vi "(notgoingtouse)ITXFolderToTDMS.vi"() -> ()   [LabVIEW 2016]
uses:
  <userlib>/LevyLab/LV to ITX/LVtoITX.lvclass
panel:
  in  "Add Values that were forgotten":T1(array[cluster])
  in  "Comment Values to say were extracted":string[](array[string])
  in  "Comment Values to extract":string[](array[string])
  in  "wave names to store (could wire to ITX->LV)":string[](array[string])
  out "Currrent ITX file":path
  in  "Ouput TDMS":path
  in  "Input ITX Folder":path=path "B:/SketchSET/SA03008H.20180718/21-BG+SG_Sweep+OVERNIGHT"
  # "Manually add values that were not recorded but are known"
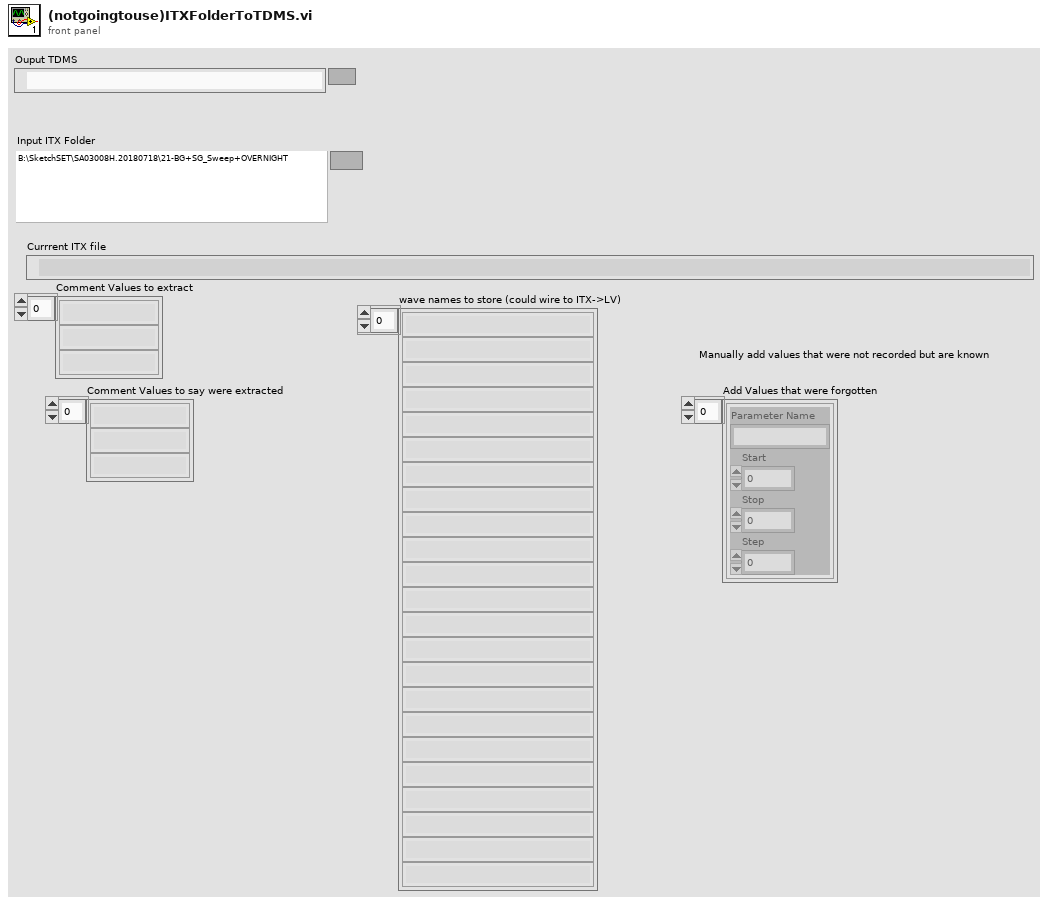
[diagram p1: front panel]
types:
  T1 = cluster{"Parameter Name":string, "Start":dbl, "Stop":dbl, "Step":dbl}[]
  T2 = enum16{"open", "open or create", "create or replace", "create", "open (read-only)"}
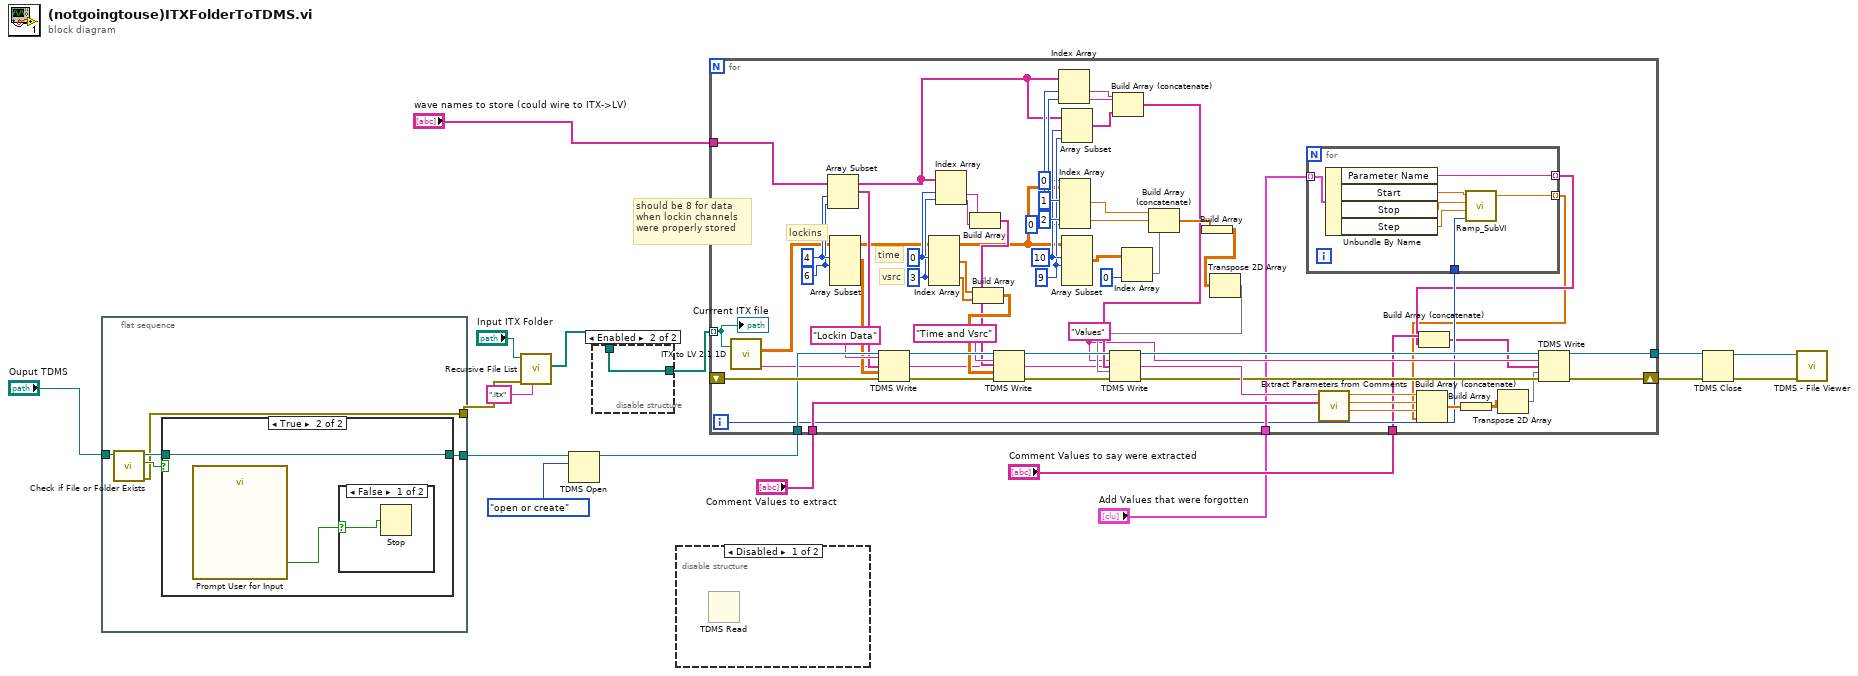
[diagram p0: block diagram]
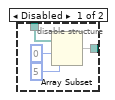
[diagram p2: hidden frame]
diagram:
  # "should be 8 for data\nwhen lockin channels\nwere properly stored"
  n1 = flat-sequence {
    tunnel: "Ouput TDMS" -> [w22]
    tunnel: [w19] -> w15
    tunnel: [w18] -> w13
    frame #0 {
      n2 = call <vilib>:"Check if File or Folder Exists.vi"("path"=w22) -> ("error out"=w18:errorcluster, "file or folder exists?"=w21:bool, "dup path"=w20:path)  [unwired: 8 in]
      n3 = case shown="True" w21 {
        tunnel: [w23 w24] -> w19
        tunnel: w20 -> [w23 w24]
        frame False {
        }
        frame True {
          n4 = call "Prompt User for Input"() -> ("Overwrite?"=w25:bool)  [unwired: 17 in, 2 out]
          n5 = case shown="False" w25 {
            selector: w25 -> [w26 _]
            frame False {
              n6 = Stop(stop? (T)=w26) -> ()
            }
            frame True {
            }
          }
        }
      }
    }
  }
  n7 = call <vilib>:"Recursive File List.vi"("pattern"=".itx", "error in (no error)"=w13, "Folder Path"="Input ITX Folder") -> ("All Files in Dir"=w7:path[])  [unwired: 4 in, 4 out]
  n8 = TDMS Open(10:T2."open or create" ("operation (0:open)"), 11:w15) -> (3:w12:refnum<k34>)  [unwired: 5 in, 1 out]
  n9 = disable-structure shown="Enabled" {
    disable-tunnel: w7 -> [w30 w31]
    disable-tunnel: [w27 w31] -> w6
    frame Disabled {
      n10 = Array Subset(array=w30, index=0, length=5) -> (w27:path[])
    }
    frame Enabled {
    }
  }
  n11 = disable-structure shown="Disabled" {
    frame Disabled {
      n12 = TDMS Read() -> ()  [unwired: 8 in, 6 out]
    }
    frame Enabled {
    }
  }
  n13 = for {
    tunnel: w6 -> [w91] mode=indexing
    tunnel: w12 -> [w89]
    tunnel: [w46] -> w11
    shift-right: [w47] -> w8
    shift-left: _ -> [w90]
    tunnel: "wave names to store (could wire to ITX->LV)" -> [w55]
    tunnel: "Comment Values to say were extracted" -> [w35]
    tunnel: "Comment Values to extract" -> [w38]
    tunnel: "Add Values that were forgotten" -> [w37]
    i -> [w36]
    w39 = "Values" ("group name in (Untitled)")
    w67 = 2 ("index (row)")
    w68 = 1 ("index (row)")
    w65 = 9 ("length")
    w66 = 10 ("index")
    w85 = 6 ("length")
    w86 = 4 ("index")
    w74 = 3 ("index (row)")
    w75 = 0 ("index (row)")
    # "lockins"
    # "vsrc"
    # "time"
    n14 = call <userlib>:"ITX to LV 2.1 1D.vi"("file (use dialog)"=w91) -> ("1D arrays"=w59:dbl[][], "Notes"=w50:string)  [unwired: 2 in, 1 out]
    n15 = Array Subset(array=w55, index=w86, length=w85) -> (w84:string[])
    n16 = Array Subset(array=w59, index (row)=w86, length (row)=w85) -> (w87:dbl[][])  [unwired: 2 in]
    n17 = TDMS Write(0:w89, 5:"Lockin Data" ("group name in (Untitled)"), 7:w84, 9:w87, 11:w90) -> (4:w82:refnum<k34>, 15:w83:errorcluster)  [unwired: 1 in, 2 out]
    n18 = Index Array(array=w59, index (row) #1=w75, index (row) #2=w74) -> (element #1=w80:dbl[], element #2=w79:dbl[])  [unwired: 2 in]
    n19 = Index Array(array=w55, index #1=w75, index #2=w74) -> (element #1=w73:string, element #2=w72:string)
    n20 = Build Array(w73, w72) -> (w71:string[])
    n21 = Build Array(w80, w79) -> (w78:dbl[][])
    n22 = TDMS Write(0:w82, 5:"Time and Vsrc" ("group name in (Untitled)"), 7:w71, 9:w78, 11:w83) -> (4:w76:refnum<k34>, 15:w77:errorcluster)  [unwired: 1 in, 2 out]
    n23 = Index Array(array=w55, index #1=w68, index #2=w67) -> (element #1=w64:string, element #2=w63:string)
    n24 = Index Array(array=w59, index (row) #1=w68, index (col) #1=0 ("disabled index (col)"), index (row) #2=w67, index (col) #2=0 ("disabled index (col)")) -> (element #1=w70:dbl, element #2=w69:dbl)
    n25 = Array Subset(array=w55, index=w66, length=w65) -> (w62:string[])
    n26 = Array Subset(array=w59, index (row)=w66, length (row)=w65) -> (w58:dbl[][])  [unwired: 2 in]
    n27 = Build Array (concatenate)(w64, w63, w62) -> (w53:string[])
    n28 = Index Array(array=w58, index (col)=0 ("disabled index (col)")) -> (element=w56:dbl[])  [unwired: 1 in]
    n29 = Build Array (concatenate)(w70, w69, w56) -> (w54:dbl[])
    n30 = Build Array(w54) -> (w52:dbl[][])
    n31 = Transpose 2D Array(2D array=w52) -> (transposed array=w51:dbl[][])
    n32 = TDMS Write(0:w76, 5:w39, 7:w53, 9:w51, 11:w77) -> (4:w49:refnum<k34>, 15:w48:errorcluster)  [unwired: 1 in, 2 out]
    n33 = for {
      tunnel: w37 -> [w98] mode=indexing
      tunnel: w36 -> [w94]
      tunnel: [w93] -> w34 mode=indexing
      tunnel: [w92] -> w32 mode=indexing
      n34 = Unbundle By Name(w98) -> ("Parameter Name"=w93:string, "Start"=w97:dbl, "Stop"=w96:dbl, "Step"=w95:dbl)
      n35 = call <userlib>:"Ramp_SubVI.vi"("index"=w94, "step"=w95, "end"=w96, "start"=w97) -> ("Numeric"=w92:dbl)  [unwired: 1 in, 1 out]
    }
    n36 = call <userlib>:"Extract Parameters from Comments.vi"("Scan names"=w38, "Comments"=w50) -> ("Numeric"=w43:dbl, "Numeric 3"=w44:dbl, "Numeric 2"=w45:dbl)  [unwired: 7 in]
    n37 = Build Array (concatenate)(w45, w44, w43, w32) -> (w40:dbl[])
    n38 = Build Array (concatenate)(w35, w34) -> (w33:string[])
    n39 = Build Array(w40) -> (w42:dbl[][])
    n40 = Transpose 2D Array(2D array=w42) -> (transposed array=w41:dbl[][])
    n41 = TDMS Write(0:w49, 5:w39, 7:w33, 9:w41, 11:w48) -> (4:w46:refnum<k34>, 15:w47:errorcluster)  [unwired: 1 in, 2 out]
    "Currrent ITX file" <- w91
  }
  n42 = TDMS Close(8:w8, 11:w11) -> (0:w9:errorcluster, 3:w10:path)
  n43 = call <vilib>:"TDMS - File Viewer.vi"("error in (no error)"=w9, "file path"=w10) -> ()  [unwired: 4 in, 2 out]
